vi "RELAYS Write the Dev Addr.vi"(8 "error in (no error)":errorcluster, 10 "Dev Addr":u8=1, 11 "VISA resource name":refnum<visa-resource-name>) -> (0 "error out":errorcluster, 1 "written Address":u8, 2 "ack":string, 3 "VISA resource name out":refnum<visa-resource-name>)   [LabVIEW 2016, in "MB _relays.lvlib"]
uses:
  MB _relays.lvlib
  private/gen MB frame -Set the device address.vi
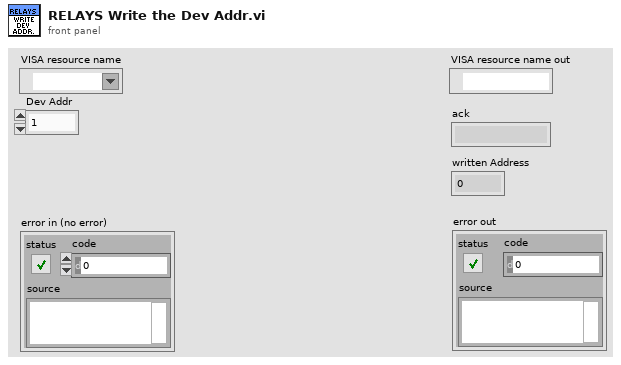
[diagram p1: front panel]
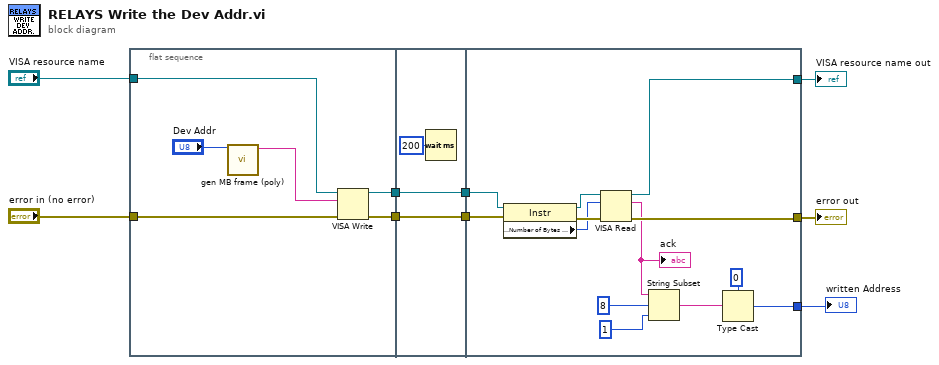
[diagram p0: block diagram]
diagram:
  n1 = flat-sequence {
    tunnel: "error in (no error)" -> [w12]
    tunnel: "VISA resource name" -> [w11]
    tunnel: [w15] -> w5
    tunnel: [w14] -> w4
    tunnel: w5 -> [w18]
    tunnel: w4 -> [w17]
    tunnel: [w18] -> w3
    tunnel: [w17] -> w2
    tunnel: [w25] -> w8
    tunnel: [w26] -> w9
    tunnel: w3 -> [w30]
    tunnel: w2 -> [w31]
    tunnel: [w19] -> w1
    frame #0 {
      n2 = call-poly "gen MB frame (poly).vi"("Dev Addr"="Dev Addr") -> ("MB frame"=w13:string)  [unwired: 10 in]
      n3 = VISA Write(VISA resource name=w11, write buffer=w13, error in (no error)=w12) -> (VISA resource name out=w15:refnum<visa-resource-name>, error out=w14:errorcluster)  [unwired: 1 out]
    }
    frame #1 {
      n4 = Wait (ms)(milliseconds to wait=u32 200) -> ()  [unwired: 1 out]
    }
    frame #2 {
      n5 = property class="Instr"(reference=w30, error in=w31) -> (reference out=w28:refnum<visa-resource-name>, error out=w29:errorcluster, "Serial Settings:Number of Bytes at Serial Port"=w27:u32)
      n6 = VISA Read(VISA resource name=w28, byte count=w27, error in (no error)=w29) -> (VISA resource name out=w26:refnum<visa-resource-name>, read buffer=w20:string, error out=w25:errorcluster)  [unwired: 1 out]
      "ack" <- w20
      n7 = String Subset(string=w20, offset (0)=8, length (rest)=1 ("length (rest)")) -> (substring=w23:string)
      n8 = Type Cast(type=u8 0, x=w23) -> (*(type *) &x=w19:u8)
    }
  }
  "VISA resource name out" <- w9
  "error out" <- w8
  "written Address" <- w1
